vi "CAL-Create Stimulus.vi"(0 "Cal Stimulus":T1={"Type"="", "Freq step (Hz)"=50.0, "Sampling rate (Hz)"=50000.0, "Attenuation (dB)"=20.0}, 11 "error in (no error)":errorcluster) -> (4 "Stimulus":dbl[](array[numeric]), 15 "error out":errorcluster)   [LabVIEW 2020]
uses:
  Typedefs/CAL-Stimulus.ctl
  a270ac18-0af9-4dde-891f-38f00d703c3a.vi
  <vilib>/Analysis/2dsp.llb/Inverse Complex FFT.vi
  <vilib>/Analysis/NI_AALPro.lvlib
panel:
  out "Phase graph":cluster{i32, "Freq Step (Hz)":dbl, dbl[]}(graph)
  out "Magnitude graph":cluster{i32, "Freq Step (Hz)":dbl, dbl[]}(graph)
  out "Signal graph":cluster{i32, dbl, dbl[]}(graph)
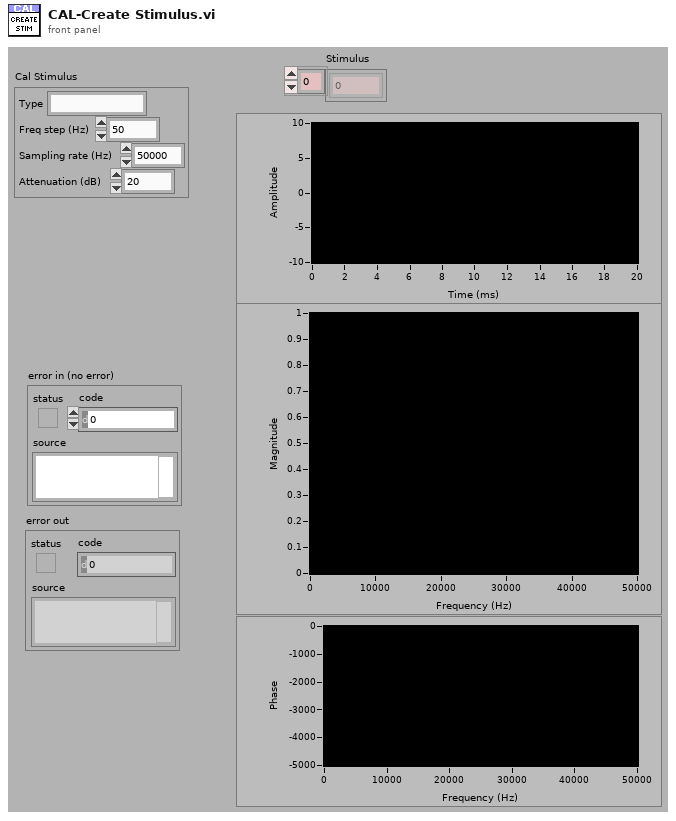
[diagram p1: front panel]
types:
  T1 = typedef "CAL-Stimulus.ctl" = cluster{"Type":string, "Freq step (Hz)":dbl, "Sampling rate (Hz)":dbl, "Attenuation (dB)":dbl}
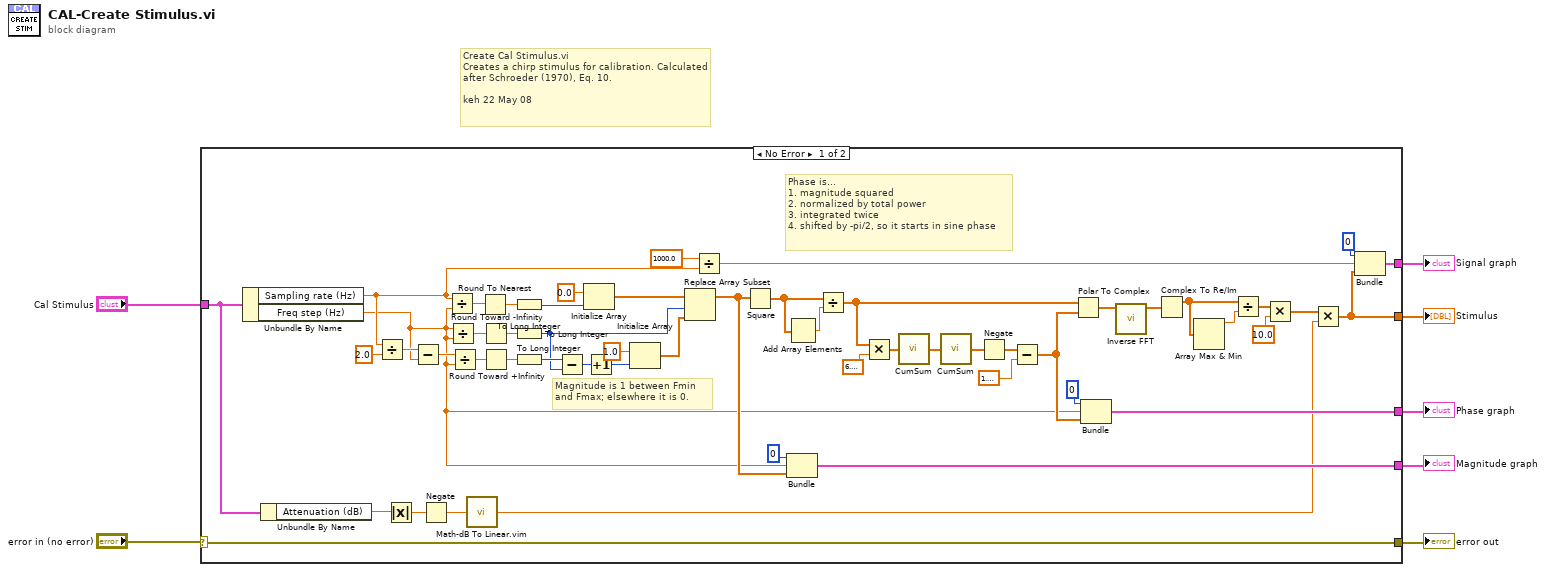
[diagram p0: block diagram]
diagram:
  # "Create Cal Stimulus.vi\nCreates a chirp stimulus for calibration. Calculated after Schroeder (1970), Eq. 10.\n\nkeh 22 May 08"
  n1 = case shown="No Error" "error in (no error)" {
    selector: "error in (no error)" -> [w22 w61]
    tunnel: "Cal Stimulus" -> [w12 _]
    tunnel: [w60 _] -> w7
    tunnel: [w59 _] -> w6
    tunnel: [w58 _] -> w5
    tunnel: [w13 _] -> w1
    tunnel: [w22 w61] -> w2
    frame No Error {
      # "Phase is...\n1. magnitude squared\n2. normalized by total power\n3. integrated twice\n4. shifted by -pi/2, so it starts in sine phase"
      # "Magnitude is 1 between Fmin\nand Fmax; elsewhere it is 0."
      n2 = Unbundle By Name(w12) -> ("Sampling rate (Hz)"=w16:dbl, "Freq step (Hz)"=w14:dbl)
      n3 = Unbundle By Name(w12) -> ("Attenuation (dB)"=w11:dbl)
      n4 = Divide(x=w16, y=2.0) -> (x/y=w17:dbl)
      n5 = Absolute Value(x=w11) -> (abs(x)=w10:dbl)
      n6 = Subtract(x=w17, y=w14) -> (x-y=w18:dbl)
      n7 = Negate(x=w10) -> (-x=w9:dbl)
      n8 = Divide(x=w16, y=w14) -> (x/y=w56:dbl)
      n9 = Divide(x=w14, y=w14) -> (x/y=w52:dbl)
      n10 = Divide(x=w18, y=w14) -> (x/y=w51:dbl)
      n11 = call "Math-dB To Linear.vim"("dB"=w9) -> ("linear"=w8:dbl)
      n12 = Round To Nearest(number=w56) -> (nearest integer value=w55:dbl)
      n13 = Round Toward -Infinity(1:w52) -> (0:w49:dbl)
      n14 = Round Toward +Infinity(x=w51) -> (ceil(x): smallest int >= x=w50:dbl)
      n15 = To Long Integer(number=w55) -> (32bit integer=w54:i32)
      n16 = To Long Integer(number=w49) -> (32bit integer=w45:i32)
      n17 = To Long Integer(number=w50) -> (32bit integer=w46:i32)
      n18 = Subtract(x=w46, y=w45) -> (x-y=w44:i32)
      n19 = Initialize Array(0.0 ("element"), w54) -> (w48:dbl[])
      n20 = Increment(x=w44) -> (x+1=w43:i32)
      n21 = Initialize Array(1.0 ("element"), w43) -> (w42:dbl[])
      n22 = Replace Array Subset(array=w48, new element=w42, index=w45) -> (w40:dbl[])
      n23 = Divide(x=1000.0, y=w16) -> (x/y=w24:dbl)
      n24 = Square(x=w40) -> (x^2=w39:dbl[])
      n25 = Bundle(0, "Freq step (Hz)"=w14, w40) -> (w60:cluster{i32, "Freq step (Hz)":dbl, dbl[]})  [unwired: 1 in]
      n26 = Add Array Elements(numeric array=w39) -> (sum=w38:dbl)
      n27 = Divide(x=w39, y=w38) -> (x/y=w32:dbl[])
      n28 = Multiply(x=w32, y=6.283185307179586) -> (x*y=w36:dbl[])
      n29 = call "CumSum.vi"("Array"=w36) -> ("CumSum"=w35:dbl[])
      n30 = call "CumSum.vi"("Array"=w35) -> ("CumSum"=w34:dbl[])
      n31 = Negate(x=w34) -> (-x=w29:dbl[])
      n32 = Subtract(x=w29, y=1.5707963267948966) -> (x-y=w28:dbl[])
      n33 = Polar To Complex(1:w28, 2:w32) -> (0:w31:cdb[])
      n34 = Bundle(0, "Freq step (Hz)"=w14, w28) -> (w59:cluster{i32, "Freq step (Hz)":dbl, dbl[]})  [unwired: 1 in]
      n35 = call-poly <vilib>:"Inverse FFT.vi"("FFT {X}"=w31) -> ("X"=w30:cdb[])  [unwired: 9 in, 1 out]
      n36 = Complex To Re/Im(x + iy=w30) -> (x=w23:dbl[])  [unwired: 1 out]
      n37 = Array Max & Min(array=w23) -> (max value=w21:dbl)  [unwired: 3 out]
      n38 = Divide(x=w23, y=w21) -> (x/y=w20:dbl[])
      n39 = Multiply(x=w20, y=10.0) -> (x*y=w57:dbl[])
      n40 = Multiply(x=w57, y=w8) -> (x*y=w13:dbl[])
      n41 = Bundle(0, w24, w13) -> (w58:cluster{i32, dbl, dbl[]})  [unwired: 1 in]
    }
    frame Error {
    }
  }
  "Stimulus" <- w1
  "Signal graph" <- w5
  "Magnitude graph" <- w7
  "Phase graph" <- w6
  "error out" <- w2
